vi "set UIVIname.vi"(8 "error in (no error)":errorcluster, 10 "UI VI name":string, 11 "xceDataNode in":refnum<class "xceDataNode.lvclass">) -> (0 "error out":errorcluster, 3 "xceDataNode out":refnum<class "xceDataNode.lvclass">)   [LabVIEW 2013, in "xceDataNode.lvclass"]
doc: "Set UIVIname. The UIVIName is the method of this class that is used to configure this node. If none is choosen, the UIVIName is mispelled, or not located in the same directory as the class, a default UI VI will be used."
uses:
  xceDataNode.lvclass
  xceDataNode.lvclass/xceDataNode.ctl
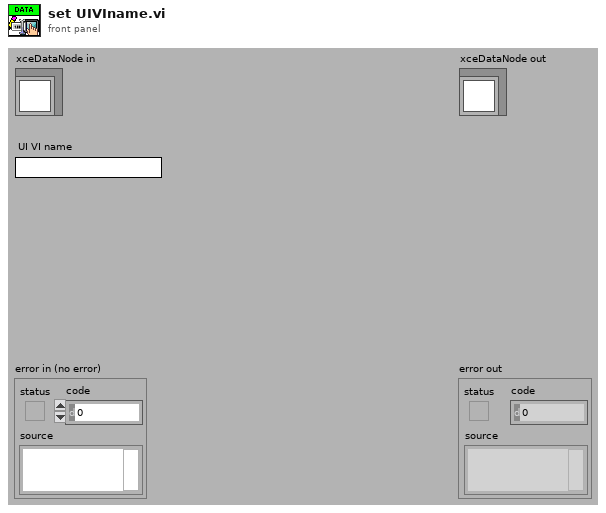
[diagram p1: front panel]
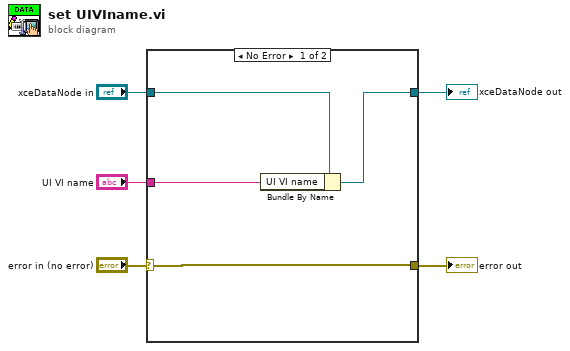
[diagram p0: block diagram]
diagram:
  n1 = case shown="No Error" "error in (no error)" {
    selector: "error in (no error)" -> [w8 w10]
    tunnel: [w8 w10] -> w1
    tunnel: [w9 w11] -> w3
    tunnel: "xceDataNode in" -> [w7 w11]
    tunnel: "UI VI name" -> [w6 _]
    frame No Error {
      n2 = Bundle By Name(cluster=w7, "UI VI name"=w6) -> (w9:refnum<class "xceDataNode.lvclass">)
    }
    frame Error {
    }
  }
  "error out" <- w1
  "xceDataNode out" <- w3
